vi "TCP-Check Result.vi"(5 "command":string, 9 "invalid response":bool, 11 "error IO":errorcluster) -> (15 "error out":errorcluster)   [LabVIEW 2020]
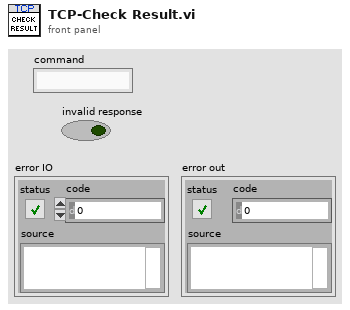
[diagram p1: front panel]
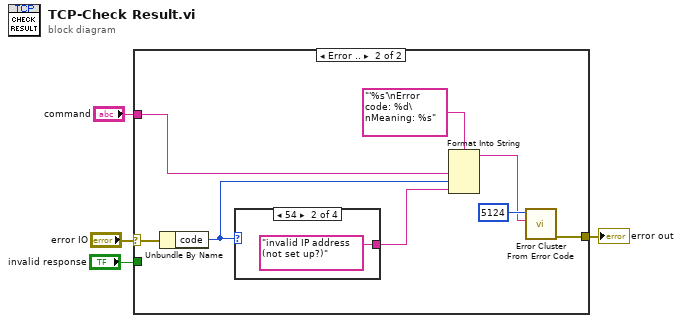
[diagram p0: block diagram]
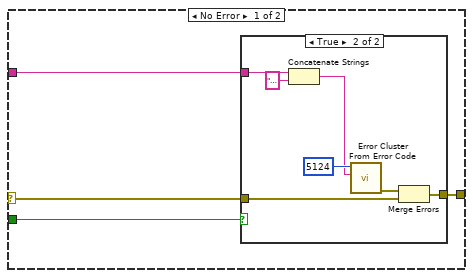
[diagram p2: hidden frame]
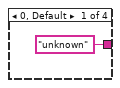
[diagram p4: hidden frame]
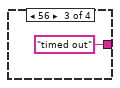
[diagram p5: hidden frame]
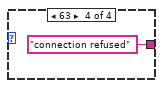
[diagram p6: hidden frame]
diagram:
  n1 = case shown="Error .." "error IO" {
    selector: "error IO" -> [w8 w22]
    tunnel: [w7 w23] -> w2
    tunnel: "invalid response" -> [w6 _]
    tunnel: "command" -> [w5 w19]
    frame No Error {
      n2 = case shown="True" w6 {
        tunnel: [w9 w14] -> w7
        tunnel: w8 -> [w9 w13]
        tunnel: w5 -> [_ w12]
        frame False {
        }
        frame True {
          n3 = Concatenate Strings(w12, " (invalid response length)" ("string")) -> (w10:string)
          n4 = call <vilib>:"Error Cluster From Error Code.vi"("error message (\"\")"=w10, "error code (0)"=5124) -> ("error out"=w16:errorcluster)  [unwired: 7 in]
          n5 = Merge Errors(w16, w13) -> (w14:errorcluster)
        }
      }
    }
    frame Error {
      n6 = Unbundle By Name(w22) -> ("code"=w18:i32)
      n7 = case shown="54" w18 {
        tunnel: ["unknown" "invalid IP address  (not set up?)" "timed out" "connection refused"] -> w17
        frame 0, Default {
        }
        frame 54 {
        }
        frame 56 {
        }
        frame 63 {
        }
      }
      n8 = Format Into String(format string="'%s'\nError code: %d\nMeaning: %s", w19, w18, w17) -> (resulting string=w20:string)  [unwired: 2 in, 1 out]
      n9 = call <vilib>:"Error Cluster From Error Code.vi"("error message (\"\")"=w20, "error code (0)"=5124) -> ("error out"=w23:errorcluster)  [unwired: 7 in]
    }
  }
  "error out" <- w2
